vi "serverfilenames.vi"(0 "Project Info":T2, 1 "Project Design Expert":T3, 7 "MathCAD results":T1, 9 "User Information":T4 {"Country" items=["Afghanistan", "Aland Islands", "Albania", "Algeria", "American Samoa", "Andorra", "Angola", "Anguilla", "Antarctica", "Antigua And Barbuda", "Argentina", "Armenia", "Aruba", "Australia", "Austria", "Azerbaijan", "Bahamas", "Bahrain", "Bangladesh", "Barbados", "Belarus", "Belgium", "Belize", "Benin", "Bermuda", "Bhutan", "Bolivia", "Bosnia And Herzegovina", "Botswana", "Bouvet Island", "Brazil", "British Indian Ocean Territory", "Brunei Darussalam", "Bulgaria", "Burkina Faso", "Burundi", "Cambodia", "Cameroon", "Canada", "Cape Verde", "Cayman Islands", "Central African Republic", "Chad", "Chile", "China", "Christmas Island", "Cocos (Keeling) Islands", "Colombia", "Comoros", "Congo", "Congo, The Democratic Republic Of The", "Cook Islands", "Costa Rica", "Cote D'Ivoire", "Croatia", "Cuba", "Cyprus", "Czech Republic", "Denmark", "Djibouti", "Dominica", "Dominican Republic", "Ecuador", "Egypt", "El Salvador", "Equatorial Guinea", "Eritrea", "Estonia", "Ethiopia", "Falkland Islands (Malvinas)", "Faroe Islands", "Fiji", "Finland", "France", "French Guiana", "French Polynesia", "French Southern Territories", "Gabon", "Gambia", "Georgia", "Germany", "Ghana", "Gibraltar", "Greece", "Greenland", "Grenada", "Guadeloupe", "Guam", "Guatemala", "Guernsey", "Guinea", "Guinea-Bissau", "Guyana", "Haiti", "Heard Island And Mcdonald Islands", "Holy See (Vatican City State)", "Honduras", "Hong Kong", "Hungary", "Iceland", "India", "Indonesia", "Iran, Islamic Republic Of", "Iraq", "Ireland", "Isle Of Man", "Israel", "Italy", "Jamaica", "Japan", "Jersey", "Jordan", "Kazakhstan", "Kenya", "Kiribati", "Korea, Democratic People'S Republic Of", "Korea, Republic Of", "Kuwait", "Kyrgyzstan", "Lao People'S Democratic Republic", "Latvia", "Lebanon", "Lesotho", "Liberia", "Libyan Arab Jamahiriya", "Liechtenstein", "Lithuania", "Luxembourg", "Macao", "Macedonia, The Former Yugoslav Republic Of", "Madagascar", "Malawi", "Malaysia", "Maldives", "Mali", "Malta", "Marshall Islands", "Martinique", "Mauritania", "Mauritius", "Mayotte", "Mexico", "Micronesia, Federated States Of", "Moldova, Republic Of", "Monaco", "Mongolia", "Montserrat", "Morocco", "Mozambique", "Myanmar", "Namibia", "Nauru", "Nepal", "Netherlands", "Netherlands Antilles", "New Caledonia", "New Zealand", "Nicaragua", "Niger", "Nigeria", "Niue", "Norfolk Island", "Northern Mariana Islands", "Norway", "Oman", "Pakistan", "Palau", "Palestinian Territory, Occupied", "Panama", "Papua New Guinea", "Paraguay", "Peru", "Philippines", "Pitcairn", "Poland", "Portugal", "Puerto Rico", "Qatar", "Reunion", "Romania", "Russian Federation", "Rwanda", "Saint Helena", "Saint Kitts And Nevis", "Saint Lucia", "Saint Pierre And Miquelon", "Saint Vincent And The Grenadines", "Samoa", "San Marino", "Sao Tome And Principe", "Saudi Arabia", "Senegal", "Serbia And Montenegro", "Seychelles", "Sierra Leone", "Singapore", "Slovakia", "Slovenia", "Solomon Islands", "Somalia", "South Africa", "South Georgia And The South Sandwich Islands", "Spain", "Sri Lanka", "Sudan", "Suriname", "Svalbard And Jan Mayen", "Swaziland", "Sweden", "Switzerland", "Syrian Arab Republic", "Taiwan, Province Of China", "Tajikistan", "Tanzania, United Republic Of", "Thailand", "Timor-Leste", "Togo", "Tokelau", "Tonga", "Trinidad And Tobago", "Tunisia", "Turkey", "Turkmenistan", "Turks And Caicos Islands", "Tuvalu", "Uganda", "Ukraine", "United Arab Emirates", "United Kingdom", "United States", "United States Minor Outlying Islands", "Uruguay", "Uzbekistan", "Vanuatu", "Venezuela", "Viet Nam", "Virgin Islands, British", "Virgin Islands, U.S.", "Wallis And Futuna", "Western Sahara", "Yemen", "Zambia", "Zimbabwe", "(Not Specified)"]}, 11 "error in (no error)":errorcluster, 12 "Project command":T6=enum."New project", 13 "Good design":bool) -> (4 "File paths":T8, 6 "attachments":T7(array[cluster]), 8 "File List":string[](array[string]), 10 "Project Info out":T2, 15 "error out":errorcluster)   [LabVIEW 2015]
uses:
  <vilib>/Utility/SMTP/NI_SMTPEmail.lvlib
  AguaClara Library.lvlib
  Folders.ctl
  Project inputs.ctl
  File paths.ctl
  Project commands.ctl
  User Information.ctl
  MathCAD results ref.ctl
  user project design.ctl
  Country Ring.ctl
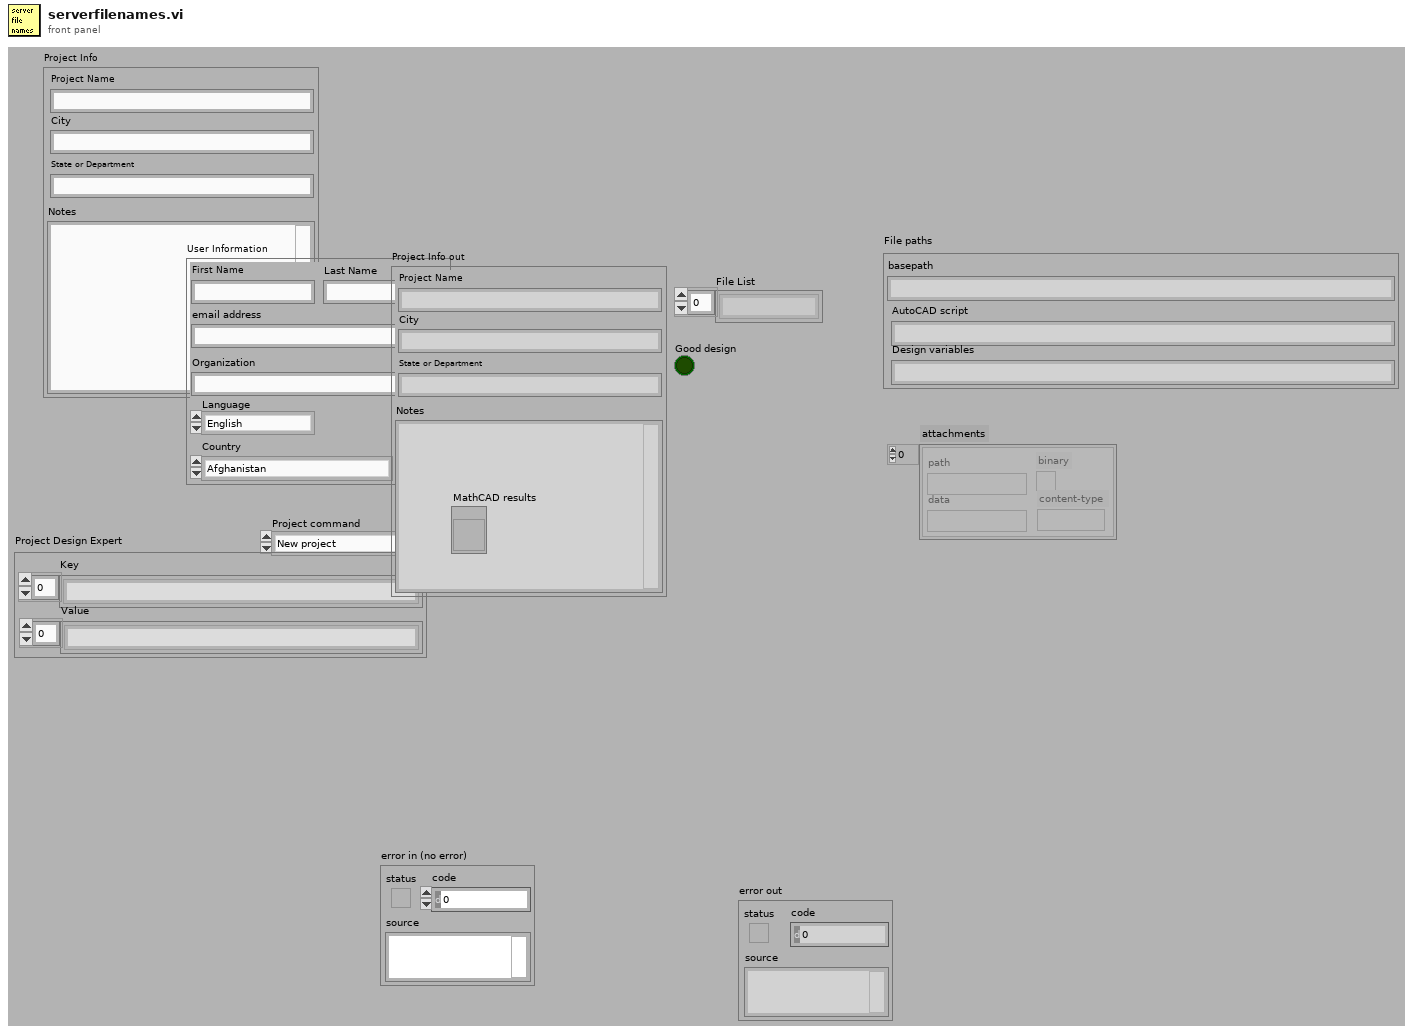
[diagram p1: front panel]
types:
  T1 = typedef "MathCAD results ref.ctl" = refnum<vi>
  T2 = typedef "AguaClara Library.lvlib/Project inputs.ctl" = cluster{"Project Name":string, "City":string, "State":string, "Notes":string}
  T3 = typedef "user project design.ctl" = cluster{"Key":string[], "Value":string[]}
  T4 = typedef "AguaClara Library.lvlib/User Information.ctl" = cluster{"First Name":string, "Last Name":string, "Email Address":string, "Organization":string, "Language":enum16{"English", "Español", "French"}, "Country":T5}
  T5 = typedef "Country Ring.ctl" = u16
  T6 = typedef "AguaClara Library.lvlib/Project commands.ctl" = enum16{"Load base file", "Load User", "Read paths", "Open Project", "New project", "Edit project", "Delete project", "Mail project", "save design", "open design"}
  T7 = cluster{"path":path, "data":string, "binary":bool, "content-type":string}[]
  T8 = typedef "AguaClara Library.lvlib/File paths.ctl" = cluster{"basepath":string, "AutoCAD script":string, "Design variables":string}
  T9 = typedef "Folders.ctl" = enum16{"DesignTool", "RequestedDesigns", "CompletedDesigns"}
  T10 = enum16{"open", "replace", "create", "open or create", "replace or create", "replace or create with confirmation"}
  T11 = typedef "AguaClara Library.lvlib/Basic Inputs.ctl" = cluster{"Q.Plant":dbl[unit], "C.CoagDoseMax":dbl[unit], "C.CoagStock":dbl[unit], "Ti.CoagStock":dbl[unit], "EN.DrillSeries":enum16{"English", "Metric"}, "EN.TubeSeries":enum16{"English", "Metric"}, "N.SedTanks":dbl, "N.SedBaysEst":dbl, "W.SedPlate":dbl[unit], "L.SedPlateSheet":dbl[unit], "T.SedPlate":dbl[unit], "T.PlantWall":dbl[unit], "H.FlocOption":dbl[unit], "T.FlocBaffleRigidH":dbl[unit], "T.ConcreteMin":dbl[unit], "T.SedWeir":dbl[unit], "T.FlocBaffleRigidV":dbl[unit]}
  T12 = cluster{"Label.Text":string, "Caption.Text":string[], "Control Type":u32, "Numeric":dbl, "Array":dbl[], "status":bool, "Outputs":bool[], "Str Array":string[], "String":string}[]
  T13 = cluster{"path":path, "data":string, "binary":bool, "content-type":string}
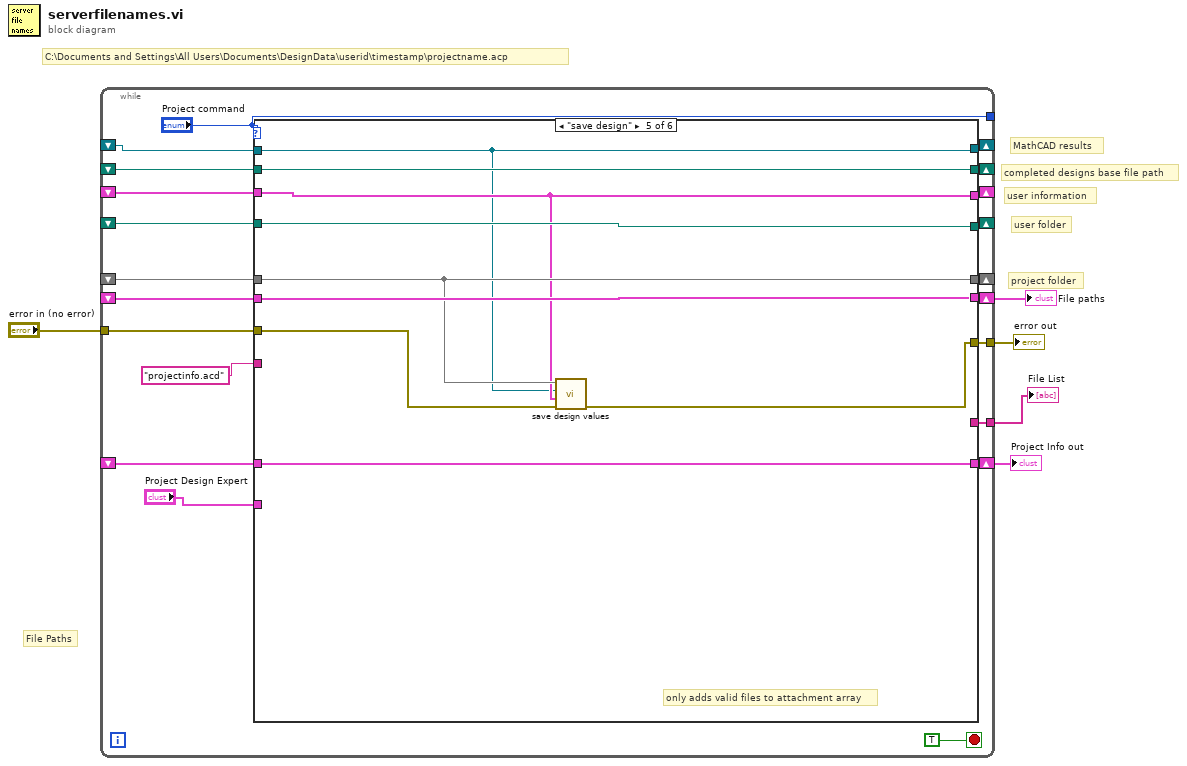
[diagram p0: block diagram]
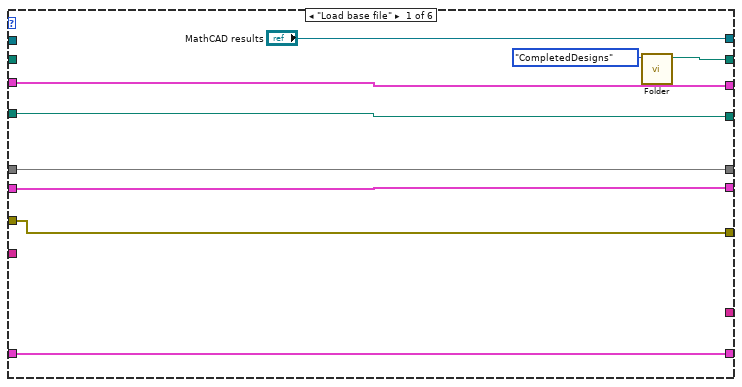
[diagram p2: hidden frame]
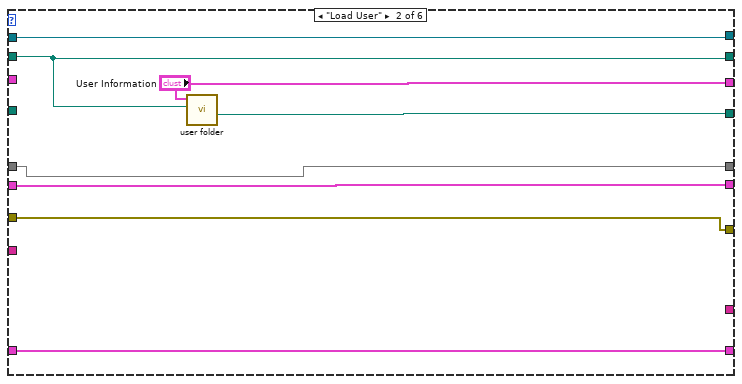
[diagram p3: hidden frame]
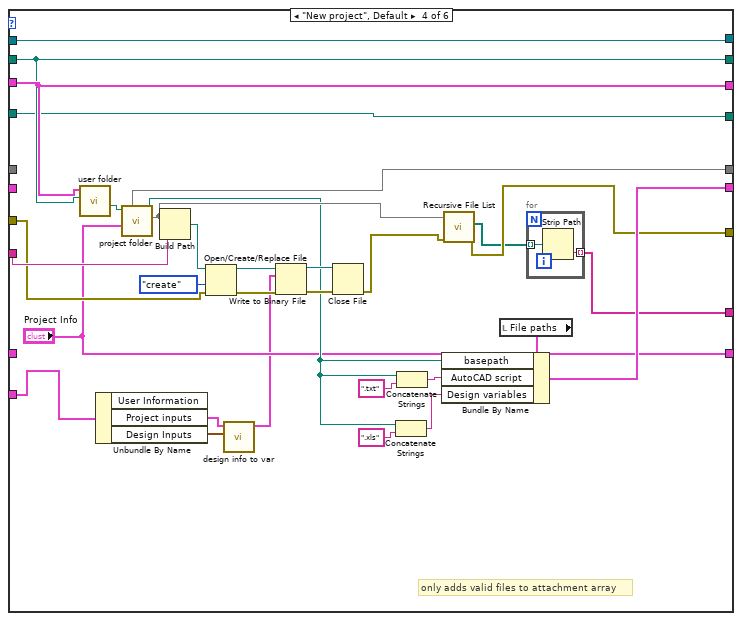
[diagram p5: hidden frame]
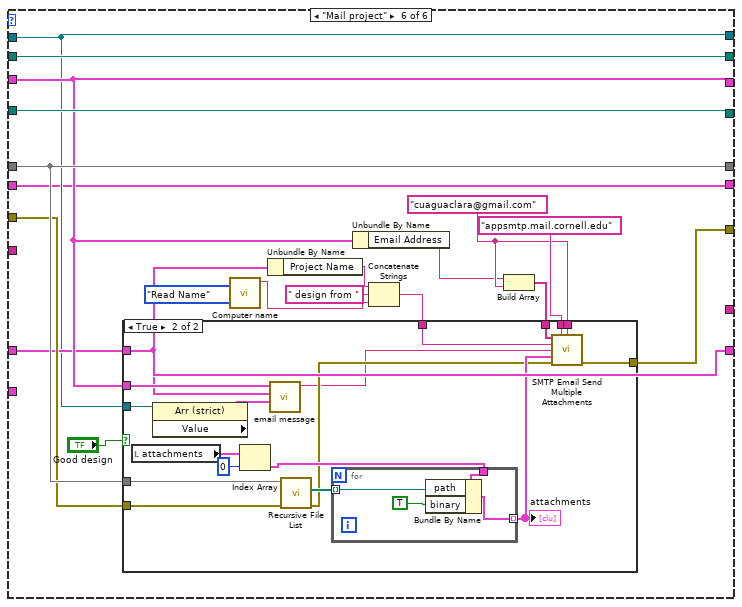
[diagram p6: hidden frame]
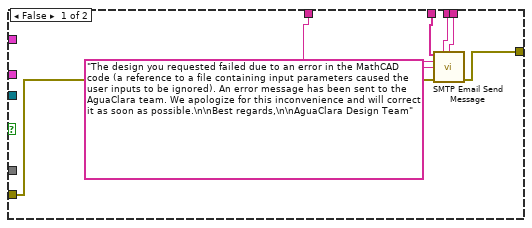
[diagram p7: hidden frame]
diagram:
  # "MathCAD results"
  # "project folder"
  # "user information"
  # "user folder"
  # "completed designs base file path"
  # "C:\\Documents and Settings\\All Users\\Documents\\DesignData\\userid\\timestamp\\projectname.acp"
  # "File Paths"
  n1 = while {
    shift-right: [w26] -> w5
    shift-left: _ -> [w25]
    shift-right: [w23] -> _
    shift-left: _ -> [w21]
    shift-right: [w22] -> _
    shift-left: _ -> [w20]
    shift-right: [w19] -> _
    shift-left: _ -> [w18]
    shift-right: [w14] -> _
    shift-left: _ -> [w13]
    tunnel: ["Project command"] -> _
    tunnel: "error in (no error)" -> [w11]
    tunnel: [w10] -> w2
    tunnel: [w9] -> w1
    shift-right: [w8] -> _
    shift-left: _ -> [w7]
    shift-right: [w16] -> w4
    shift-left: _ -> [w6]
    stop <- TRUE stop-if-true
    n2 = case shown="\"save design\"" "Project command" {
      tunnel: [w34 w43 w51 w81 w90 w94] -> w26
      tunnel: w25 -> [w34 w43 w51 _ w90 w94]
      tunnel: [w27 w41 w50 w79 w92 w111] -> w23
      tunnel: [w35 "User Information" w49 w80 w85 w102] -> w22
      tunnel: w21 -> [_ w41 w50 w79 w92 w111]
      tunnel: w20 -> [w35 _ w49 w80 w85 w102]
      tunnel: [w33 w40 w48 w78 w91 w110] -> w19
      tunnel: w18 -> [w33 _ w48 w78 w91 w110]
      tunnel: "Project Design Expert" -> [_ _ _ w55 _ _]
      tunnel: w6 -> [w32 w36 w47 _ w89 w101]
      tunnel: [w32 w36 w47 "Project Info" w89 w101] -> w16
      tunnel: "projectinfo.acd" ("name or relative path") -> [_ _ _ w77 _ _]
      tunnel: [w31 w37 w46 w76 w88 w107] -> w14
      tunnel: w13 -> [w31 w37 w46 _ w88 w107]
      tunnel: w11 -> [w30 w38 w45 w75 w87 w106]
      tunnel: [w30 w38 w45 w74 w86 w105] -> w10
      tunnel: [_ _ _ w73 _ _] -> w9
      tunnel: ["MathCAD results" w39 w44 w72 w84 w100] -> w8
      tunnel: w7 -> [_ w39 w44 w72 w84 w100]
      frame "Load base file" {
        n3 = call "Folder.vi"("Folders"=Folders."CompletedDesigns") -> ("FolderPath"=w27:path)  [unwired: 9 in, 1 out]
      }
      frame "Load User" {
        n4 = call "user folder.vi"("Base File Path"=w41, "User Information"="User Information") -> ("User folder Path"=w40:path)  [unwired: 7 in, 2 out]
      }
      frame "Read paths" {
      }
      frame "New project", Default {
        # "only adds valid files to attachment array"
        n5 = call "user folder.vi"("Base File Path"=w79, "User Information"=w80) -> ("User folder Path"=w66:path)  [unwired: 7 in, 2 out]
        n6 = Unbundle By Name(w55) -> ("Project inputs"=w54:T2, "Design Inputs"=w53:T11)  [unwired: 1 out]
        n7 = call "project folder.vi"("Request File Name"="Project Info", "Method"=w66) -> (2:w76, "Completed Design path"=w57:path)  [unwired: 7 in, 1 out]
        n8 = Build Path(base path=w76, name or relative path=w77) -> (appended path=w60:path)
        n9 = Open/Create/Replace File(file path (use dialog)=w60, error in=w75, operation (0:open)=T10."create") -> (refnum out=w63:refnum<file>, error out=w65:errorcluster)  [unwired: 3 in, 1 out]
        n10 = call "design info to var.vi"("Design Inputs"=w53, "Project Info"=w54) -> ("Array to save"=w52:cluster{"Label.Text":string, "Value":variant}[])  [unwired: 9 in]
        n11 = Write to Binary File(file (use dialog)=w63, data=w52, error in=w65) -> (refnum out=w61:refnum<file>, error out=w62:errorcluster)  [unwired: 3 in, 1 out]
        n12 = Close File(refnum=w61, error in=w62) -> (error out=w58:errorcluster)  [unwired: 1 out]
        n13 = Concatenate Strings(w57, ".xls" ("string")) -> (w67:string)
        n14 = Concatenate Strings(w57, ".txt" ("string")) -> (w70:string)
        n15 = call <vilib>:"Recursive File List.vi"("error in (no error)"=w58, "Folder Path"=w76) -> ("error out"=w74:errorcluster, "All Files in Dir"=w59:path[])  [unwired: 5 in, 3 out]
        n16 = local read "File paths"() -> (w68:T8)
        n17 = Bundle By Name(cluster=w68, "basepath"=w57, "AutoCAD script"=w70, "Design variables"=w67) -> (w81:T8)
        n18 = for {
          tunnel: w59 -> [w83] mode=indexing
          tunnel: [w82] -> w73 mode=indexing
          n19 = Strip Path(path=w83) -> (name=w82:string)  [unwired: 1 out]
        }
      }
      frame "save design" {
        # "only adds valid files to attachment array"
        n20 = call "save design values.vi"("error in"=w87, "User Information"=w85, "MathCAD results"=w84, "Project Folder"=w88) -> ("error out"=w86:errorcluster)  [unwired: 7 in]
      }
      frame "Mail project" {
        w104 = "cuaguaclara@gmail.com" ("return address")
        n21 = call "Computer name.vi"("cmd"=enum16{"Load Name", "Read Name"}."Read Name") -> ("Computer name"=w98:string)  [unwired: 9 in, 1 out]
        n22 = Unbundle By Name(w101) -> ("Project Name"=w96:string)
        n23 = Unbundle By Name(w102) -> ("Email Address"=w103:string)
        n24 = Concatenate Strings(w96, " design from " ("string"), w98) -> (w95:string)
        n25 = Build Array(w103, w104) -> (w109:string[])
        n26 = case shown="True" "Good design" {
          tunnel: w109 -> [w116 w136]
          tunnel: "appsmtp.mail.cornell.edu" ("mail server") -> [w117 w135]
          tunnel: w107 -> [_ w129]
          tunnel: w106 -> [w114 w128]
          tunnel: [w113 w126] -> w105
          tunnel: w104 -> [w118 w125]
          tunnel: w102 -> [_ w124]
          tunnel: w101 -> [_ w123]
          tunnel: w100 -> [_ w121]
          tunnel: w95 -> [w115 w119]
          frame False {
            n27 = call <vilib>:"SMTP Email Send Message.vi"("recipients"=w116, "mail server"=w117, "return address"=w118, "subject ([No Subject])"=w115, "message"="The design you requested failed due to an error in the MathCAD code (a reference to a file containing input parameters caused the user inputs to be ignored). An error message has been sent to the AguaClara team. We apologize for this inconvenience and will correct it as soon as possible.\n\nBest regards,\n\nAguaClara Design Team", "error in (no error)"=w114) -> ("error out"=w113:errorcluster)  [unwired: 8 in, 1 out]
          }
          frame True {
            n28 = local read "attachments"() -> (w134:T7)
            n29 = property class="Arr (strict)"(reference=w121) -> ("Value"=w120:T12)  [unwired: 1 in, 2 out]
            n30 = Index Array(array=w134, index=0) -> (element=w132:T13)
            n31 = call "email message.vi"("Variable Clusters"=w120, "Project Info"=w123, "User Information"=w124) -> ("Message"=w122:string)  [unwired: 8 in]
            n32 = call <vilib>:"Recursive File List.vi"("error in (no error)"=w128, "Folder Path"=w129) -> ("error out"=w127:errorcluster, "All Files in Dir"=w131:path[])  [unwired: 5 in, 3 out]
            n33 = for {
              tunnel: w131 -> [w138] mode=indexing
              tunnel: w132 -> [w140]
              tunnel: [w137] -> w130 mode=indexing
              n34 = Bundle By Name(cluster=w140, "path"=w138, "binary"=TRUE) -> (w137:T13)
            }
            "attachments" <- w130
            n35 = call <vilib>:"SMTP Email Send Multiple Attachments.vi"("recipients"=w136, "mail server"=w135, "return address"=w125, "subject ([No Subject])"=w119, "message"=w122, "attachments"=w130, "error in (no error)"=w127) -> ("error out"=w126:errorcluster)  [unwired: 7 in, 1 out]
          }
        }
      }
    }
  }
  "File paths" <- w5
  "Project Info out" <- w4
  "error out" <- w2
  "File List" <- w1
